vi "Anpassung.vi"(0 "GUI Einstellungen":T2, 1 "GUI data":T3, 2 "Globale Variablen":T1, 3 "Spg (0)":dbl=1.5 format="%#_13g", 4 "Add (0)":dbl=0.5 format="%#_13g", 5 "Error_in":errorcluster, 8 "Frequency (1000 Hz)":dbl=1000.0) -> (9 "GUI Einstellungen out":T2, 11 "GUI data out":T3, 13 "Globale Variablen out":T1, 16 "spg":dbl, 19 "Error_out":errorcluster)   [LabVIEW 2016]
uses:
  <instrlib>/Agilent 33XXX Series/Agilent 33XXX Series.lvlib
panel:
  out "i1 (wird nicht \nweiter verwendet)":i32
  out "Abbruch (VI verlassen) = merker1":bool
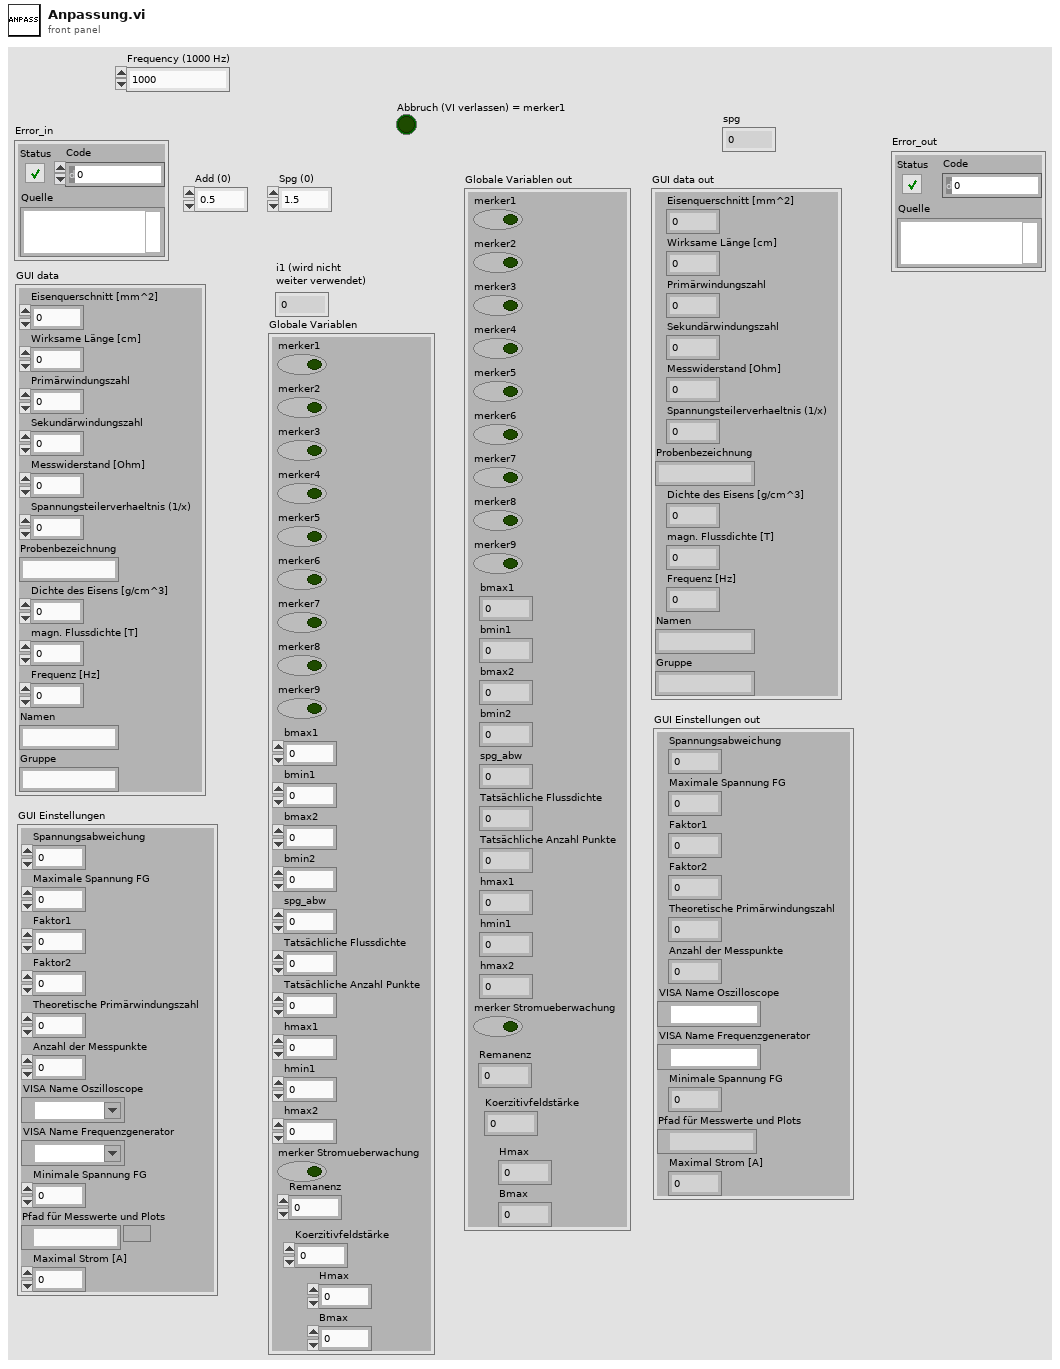
[diagram p1: front panel]
types:
  T1 = cluster{"merker1":bool, "merker2":bool, "merker3":bool, "merker4":bool, "merker5":bool, "merker6":bool, "merker7":bool, "merker8":bool, "merker9":bool, "bmax1":dbl, "bmin1":dbl, "bmax2":dbl, "bmin2":dbl, "spg_abw":dbl, "Tatsächliche Flussdichte":dbl, "Tatsächliche Anzahl Punkte":dbl, "hmax1":dbl, "hmin1":dbl, "hmax2":dbl, "merker Stromueberwachung":bool, "Remanenz":dbl, "Koerzitivfeldstärke":dbl, "Bmax":dbl, "Hmax":dbl}
  T2 = cluster{"Spannungsabweichung":dbl, "Maximale Spannung FG":dbl, "Faktor1":dbl, "Faktor2":dbl, "Theoretische Primärwindungszahl":dbl, "Anzahl der Messpunkte":i32, "VISA Name Oszilloscope":refnum<visa-resource-name>, "VISA Name Frequenzgenerator":refnum<visa-resource-name>, "Minimale Spannung FG":dbl, "Pfad für Messwerte und Plots":path, "Maximal Strom [A] ":dbl}
  T3 = cluster{"Eisenquerschnitt [mm^2]":dbl, "Wirksame Länge [cm]":dbl, "Primärwindungszahl":dbl, "Sekundärwindungszahl":dbl, "Messwiderstand [Ohm]":dbl, "Spannungsteilerverhaeltnis (1/x)":dbl, "Probenbezeichnung":string, "Dichte des Eisens [g/cm^3]":dbl, "magn. Flussdichte [T]":dbl, "Frequenz [Hz]":dbl, "Namen":string, "Gruppe":string}
  T4 = enum16{"Chk_U", "U_Einst", "Messen", "Setze merker9"}
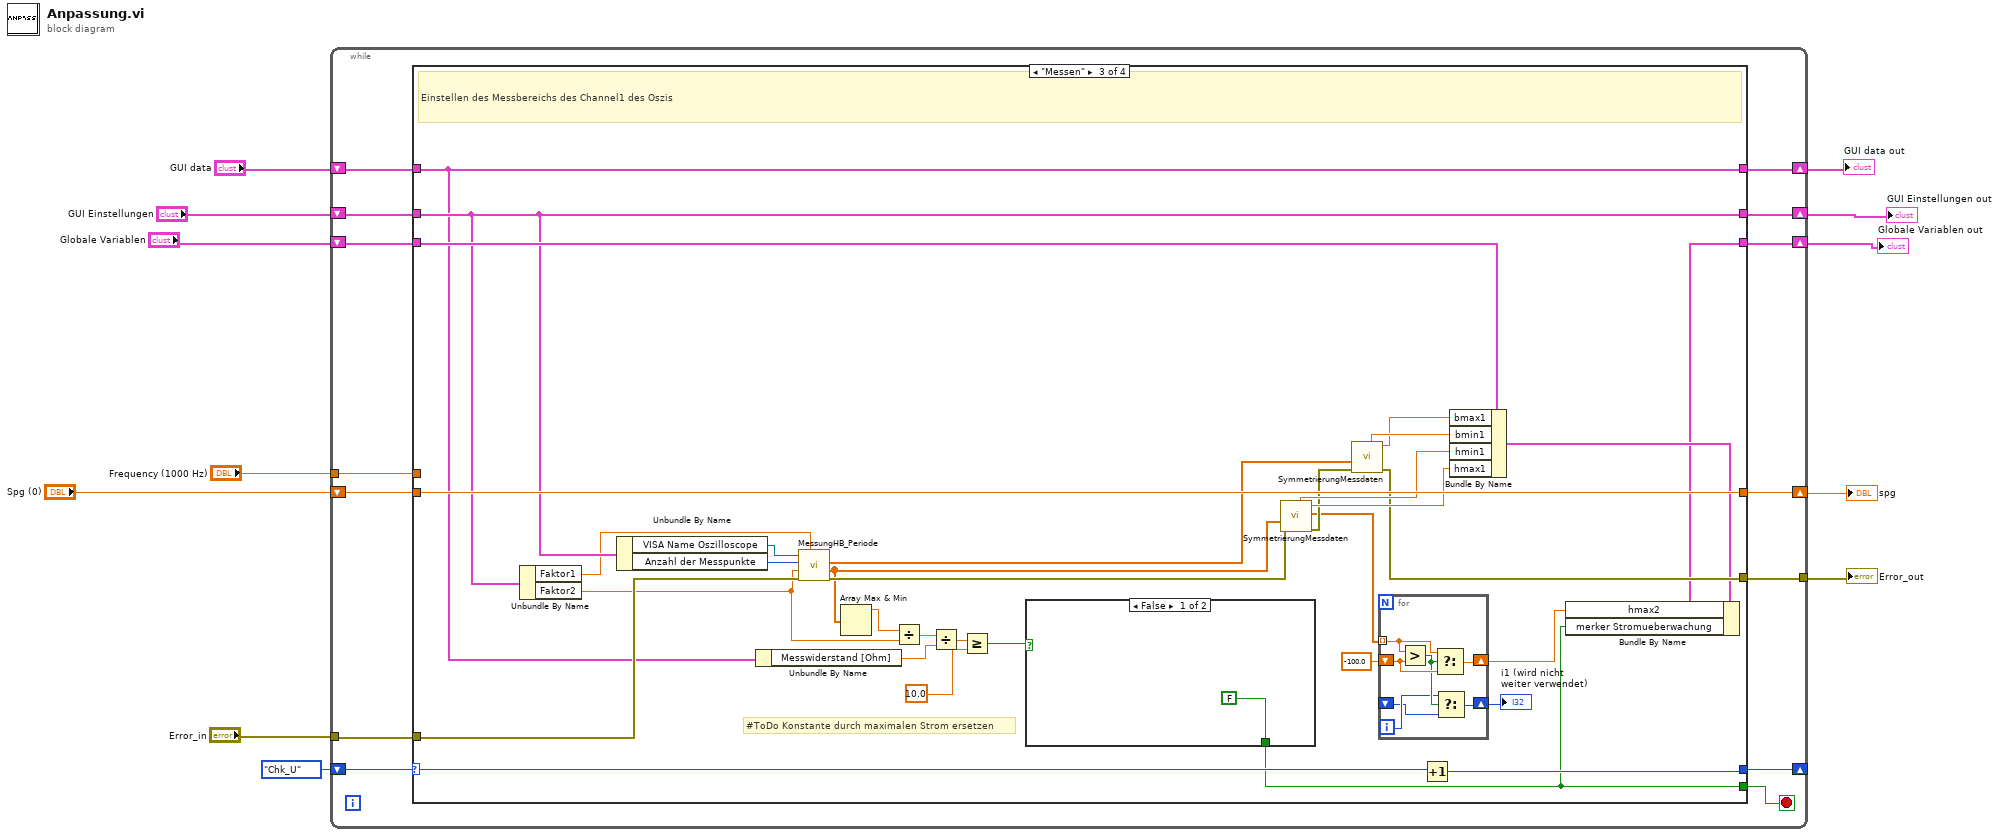
[diagram p0: block diagram]
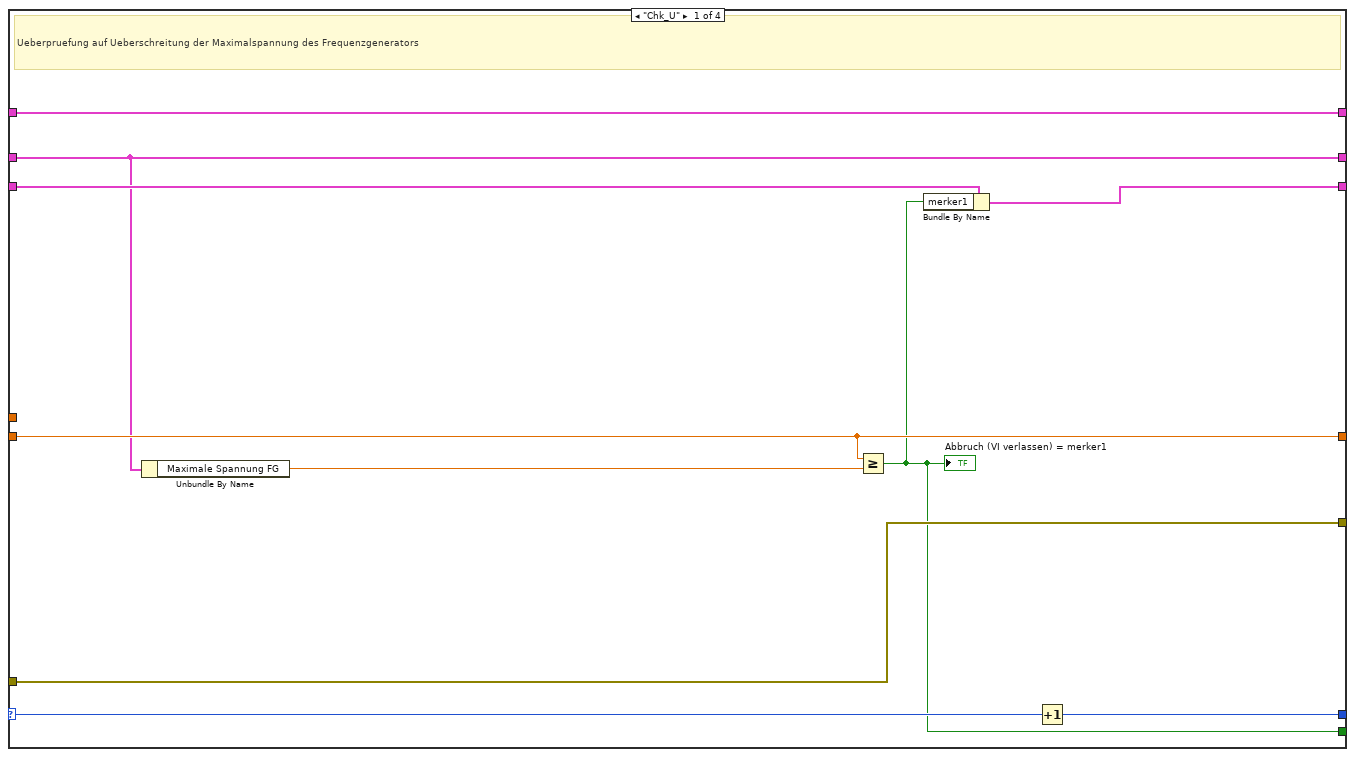
[diagram p2: hidden frame]
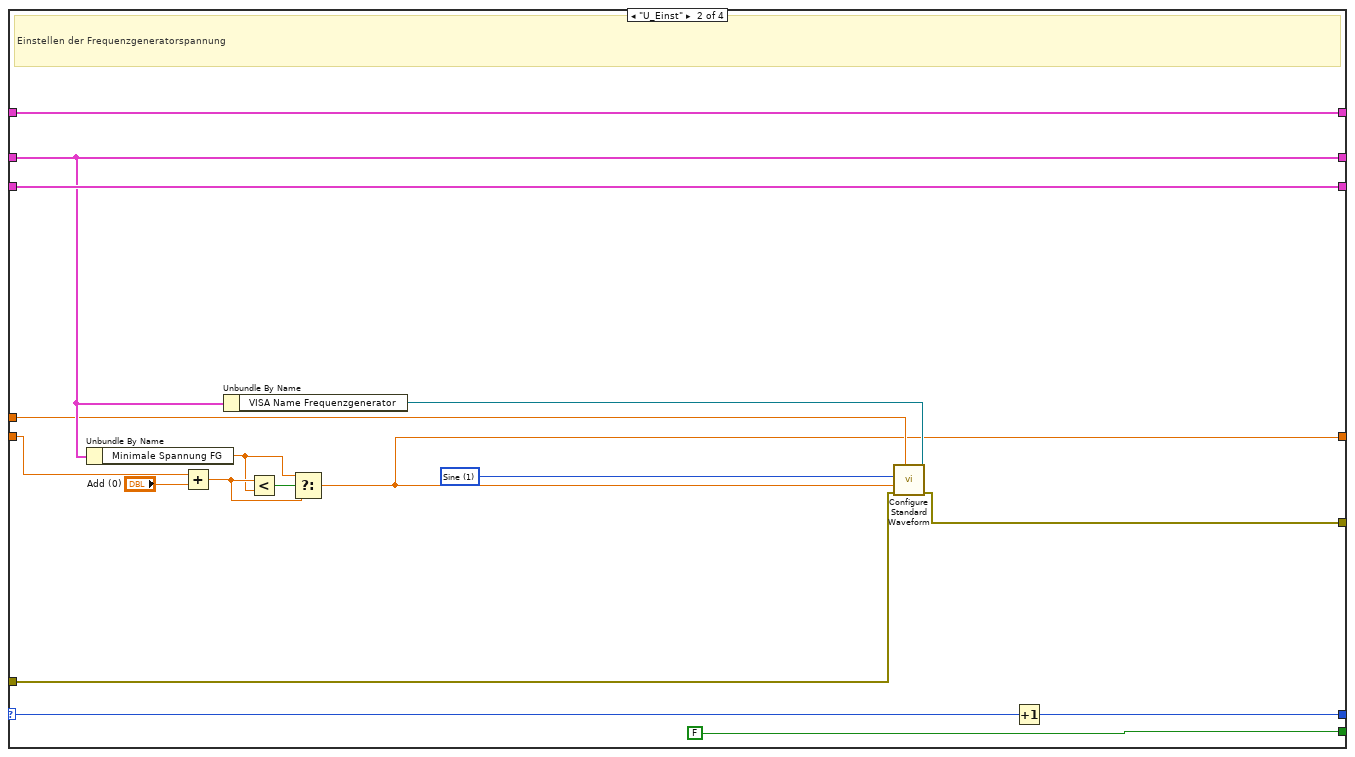
[diagram p3: hidden frame]
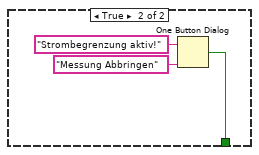
[diagram p4: hidden frame]
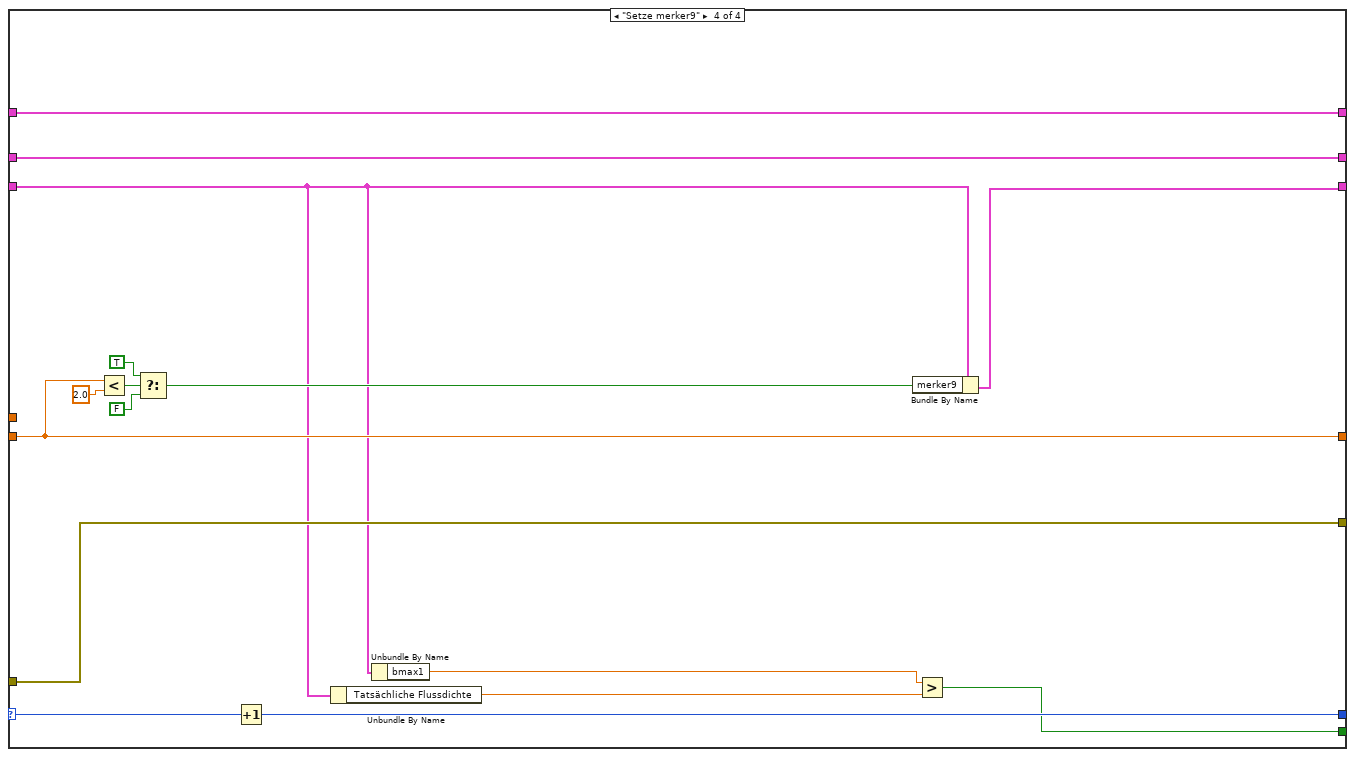
[diagram p5: hidden frame]
diagram:
  n1 = while {
    shift-right: [w26] -> _
    shift-left: T4."Chk_U" -> [w23]
    tunnel: "Error_in" -> [w25]
    tunnel: [w24] -> w11
    shift-right: [w20] -> w9
    shift-left: "Spg (0)" -> [w21]
    shift-right: [w19] -> w7
    shift-left: "GUI data" -> [w18]
    shift-right: [w16] -> w3
    shift-left: "GUI Einstellungen" -> [w17]
    shift-right: [w14] -> w1
    shift-left: "Globale Variablen" -> [w15]
    tunnel: "Frequency (1000 Hz)" -> [w13]
    stop <- w22 stop-if-true
    n2 = case shown="\"Messen\"" w23 {
      selector: w23 -> [w36 w52 w86 w104]
      tunnel: [w34 w50 w85 w103] -> w26
      tunnel: w25 -> [w35 w39 w82 w105]
      tunnel: [w35 w38 w70 w105] -> w24
      tunnel: [w29 FALSE w54 w100] -> w22
      tunnel: w21 -> [w33 w48 w84 w106]
      tunnel: [w33 w40 w84 w106] -> w20
      tunnel: [w28 w45 w59 w102] -> w19
      tunnel: w18 -> [w28 w45 w59 w102]
      tunnel: w17 -> [w27 w43 w75 w112]
      tunnel: [w27 w43 w75 w112] -> w16
      tunnel: w15 -> [w30 w44 w76 w98]
      tunnel: [w31 w44 w64 w113] -> w14
      tunnel: w13 -> [_ w42 _ _]
      frame "Chk_U" {
        # "Ueberpruefung auf Ueberschreitung der Maximalspannung des Frequenzgenerators"
        n3 = Unbundle By Name(w27) -> ("Maximale Spannung FG"=w32:dbl)
        n4 = Greater Or Equal?(x=w33, y=w32) -> (x >= y?=w29:bool)
        "Abbruch (VI verlassen) = merker1" <- w29
        n5 = Bundle By Name(cluster=w30, "merker1"=w29) -> (w31:T1)
        n6 = Increment(x=w36) -> (x+1=w34:T4)
      }
      frame "U_Einst" {
        w37 = u16 1 items=["DC", "Sine", "Square", "Triangle", "Ramp", "Pulse", "Noise", "Sinc", "Negative Ramp", "Exponential Rise", "Exponential Fall", "Cardiac"] ("Waveform Function (1: Sine)")
        # "Einstellen der Frequenzgeneratorspannung"
        n7 = Unbundle By Name(w43) -> ("Minimale Spannung FG"=w46:dbl)
        n8 = Add(x=w48, y="Add (0)") -> (x+y=w47:dbl)
        n9 = Unbundle By Name(w43) -> ("VISA Name Frequenzgenerator"=w41:refnum<visa-resource-name>)
        n10 = Less?(x=w47, y=w46) -> (x < y?=w53:bool)
        n11 = Select(t=w46, s=w53, f=w47) -> (s? t:f=w40:dbl)
        n12 = call <instrlib>:"Configure Standard Waveform.vi"("Frequency (1000 Hz)"=w42, "error in (no error)"=w39, "Amplitude (1)"=w40, "Waveform Function (1: Sine)"=w37, "VISA resource name"=w41) -> ("error out"=w38:errorcluster)  [unwired: 5 in, 1 out]
        n13 = Increment(x=w52) -> (x+1=w50:T4)
      }
      frame "Messen" {
        # "#ToDo Konstante durch maximalen Strom ersetzen"
        # "Einstellen des Messbereichs des Channel1 des Oszis"
        n14 = Unbundle By Name(w75) -> ("Faktor1"=w73:dbl, "Faktor2"=w61:dbl)
        n15 = Unbundle By Name(w75) -> ("VISA Name Oszilloscope"=w83:refnum<visa-resource-name>, "Anzahl der Messpunkte"=w74:i32)
        n16 = Unbundle By Name(w59) -> ("Messwiderstand [Ohm]"=w58:dbl)
        n17 = call "MessungHB_Periode.vi"("Faktor 1"=w73, "Error_in"=w82, "Faktor2 (1)"=w61, "Anzahl der Messpunkte"=w74, "VISA Name OZ in(OZ)"=w83) -> ("Error_out"=w72:errorcluster, "H-Messdaten einer periode"=w63:dbl[], "B-Messdaten einer periode"=w81:dbl[])  [unwired: 3 in, 1 out]
        n18 = Array Max & Min(array=w63) -> (max value=w62:dbl)  [unwired: 3 out]
        n19 = Divide(x=w62, y=w61) -> (x/y=w60:dbl)
        n20 = Divide(x=w60, y=w58) -> (x/y=w57:dbl)
        n21 = Greater Or Equal?(x=w57, y=10.0) -> (x >= y?=w55:bool)
        n22 = case shown="False" w55 {
          tunnel: [FALSE w88] -> w54
          frame False {
          }
          frame True {
            n23 = One Button Dialog(message="Strombegrenzung aktiv!" ("Nachricht"), button name ("OK")="Messung Abbringen" ("Schaltflächentext (\"OK\")")) -> (true=w88:bool)
          }
        }
        n24 = call "SymmetrierungMessdaten.vi"("error in"=w72, "Input Array"=w63) -> ("error out"=w71:errorcluster, "Output Array"=w66:dbl[], "xmax"=w77:dbl, "xmin"=w78:dbl)  [unwired: 3 in, 1 out]
        n25 = call "SymmetrierungMessdaten.vi"("error in"=w71, "Input Array"=w81) -> ("error out"=w70:errorcluster, "xmax"=w79:dbl, "xmin"=w80:dbl)  [unwired: 3 in, 2 out]
        n26 = for {
          shift-right: [w96] -> w67
          shift-left: -100.0 -> [w97]
          shift-right: [w93] -> w68
          shift-left: _ -> [w92]
          tunnel: w66 -> [w91] mode=indexing
          i -> [w94]
          n27 = Greater?(x=w91, y=w97) -> (0:w95:bool)
          n28 = Select(t=w91, s=w95, f=w97) -> (s? t:f=w96:dbl)
          n29 = Select(t=w94, s=w95, f=w92) -> (s? t:f=w93:i32)
        }
        "i1 (wird nicht \nweiter verwendet)" <- w68
        n30 = Increment(x=w86) -> (x+1=w85:T4)
        n31 = Bundle By Name(cluster=w76, "bmax1"=w79, "bmin1"=w80, "hmin1"=w78, "hmax1"=w77) -> (w65:T1)
        n32 = Bundle By Name(cluster=w65, "hmax2"=w67, "merker Stromueberwachung"=w54) -> (w64:T1)
      }
      frame "Setze merker9" {
        n33 = Less?(x=w106, y=2.0) -> (x < y?=w111:bool)
        n34 = Select(t=TRUE, s=w111, f=FALSE) -> (s? t:f=w107:bool)
        n35 = Increment(x=w104) -> (x+1=w103:T4)
        n36 = Unbundle By Name(w98) -> ("Tatsächliche Flussdichte"=w99:dbl)
        n37 = Unbundle By Name(w98) -> ("bmax1"=w101:dbl)
        n38 = Bundle By Name(cluster=w98, "merker9"=w107) -> (w113:T1)
        n39 = Greater?(x=w101, y=w99) -> (0:w100:bool)
      }
    }
  }
  "Error_out" <- w11
  "spg" <- w9
  "GUI data out" <- w7
  "GUI Einstellungen out" <- w3
  "Globale Variablen out" <- w1
